vi "Global Stop.vi"() -> ()   [LabVIEW 2015]
panel:
  in  "Global Stop":bool
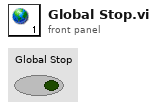
[diagram p1: front panel]
diagram:
